vi "DriveGetModuleRef.vi"(11 "ModualNamePrefix":i32) -> (0 "SpinMot":T2, 1 "SpinStr":string, 2 "TravMot":T2, 3 "TravStr":string, 4 "EncStr":string, 5 "AbsEncoder":T1)   [LabVIEW 2025]
uses:
  <vilib>/Rock Robotics/SystemInterfaces/DIO/FPGA_DIOPWMChannel.ctl
  <vilib>/Rock Robotics/WPI/PWM/WPI_PWMDeadband.ctl
  <vilib>/Rock Robotics/WPI/MotorControl/WPI_MotorControlType.ctl
  <vilib>/Rock Robotics/SystemInterfaces/DIO/FPGA_DIOChannel.ctl
  <vilib>/Rock Robotics/WPI/MotorControl/WPI_MotorControlDeviceRef.ctl
  <vilib>/Rock Robotics/WPI/ThirdParty/Phoenix6/DeviceReference.ctl
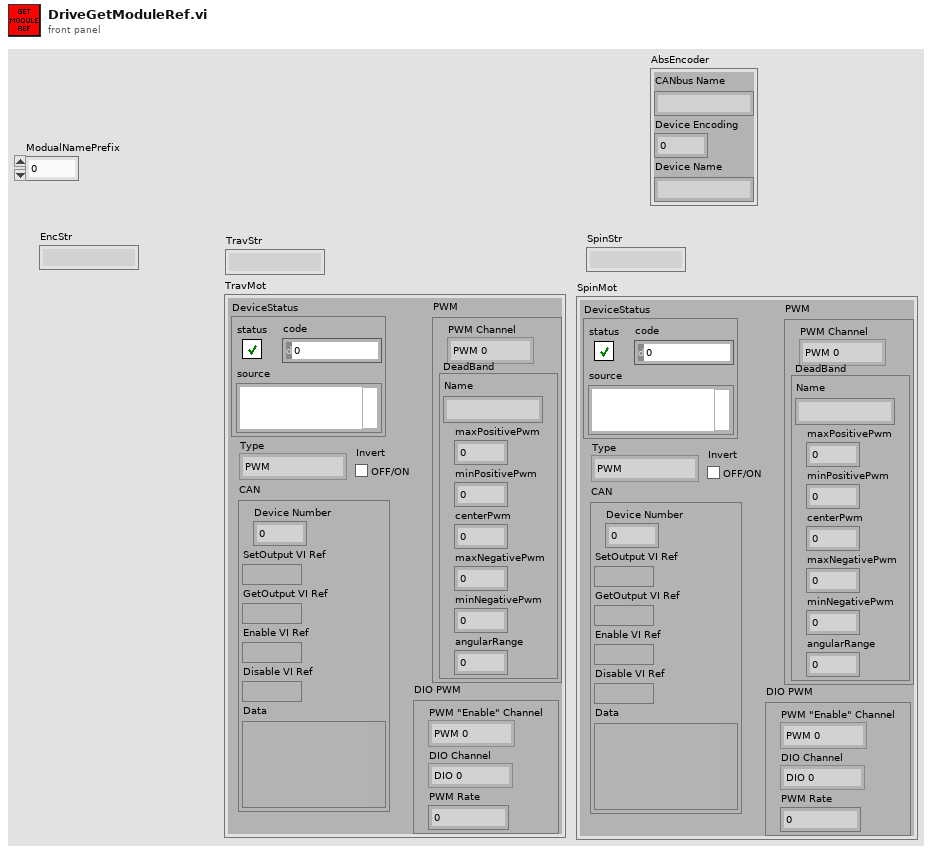
[diagram p1: front panel]
types:
  T1 = typedef "DeviceReference.ctl" = cluster{"CANbus Name":string, "Device Encoding":u32, "Device Name":string}
  T2 = typedef "WPI_MotorControlDeviceRef.ctl" = cluster{"DeviceStatus":errorcluster, "Type":T3, "PWM":cluster{"PWM Channel":T4, "DeadBand":T5}, "CAN":cluster{"Device Number":u8, "SetOutput VI Ref":variant, "GetOutput VI Ref":variant, "Enable VI Ref":variant, "Disable VI Ref":variant, "Data":variant}, "Invert":bool, "DIO PWM":cluster{"PWM \"Enable\" Channel":T4, "DIOChannel":T6, "PWM Rate":dbl}}
  T3 = typedef "WPI_MotorControlType.ctl" = enum16{"PWM", "CAN", "DIO PWM"}
  T4 = typedef "FPGA_DIOPWMChannel.ctl" = enum8{"PWM 0", "PWM 1", "PWM 2", "PWM 3", "PWM 4", "PWM 5", "PWM 6", "PWM 7", "PWM 8", "PWM 9", "PWM MXP 0", "PWM MXP 1", "PWM MXP 2", "PWM MXP 3", "PWM MXP 4", "PWM MXP 5", "PWM MXP 6", "PWM MXP 7", "PWM MXP 8", "PWM MXP 9", "Invalid"}
  T5 = typedef "WPI_PWMDeadband.ctl" = cluster{"Name":string, "maxPositivePwm":i32, "minPositivePwm":i32, "centerPwm":i32, "maxNegativePwm":i32, "minNegativePwm":i32, "angularRange":u16}
  T6 = typedef "FPGA_DIOChannel.ctl" = enum8{"DIO 0", "DIO 1", "DIO 2", "DIO 3", "DIO 4", "DIO 5", "DIO 6", "DIO 7", "DIO 8", "DIO 9", "DIO MXP 0", "DIO MXP 1", "DIO MXP 2", "DIO MXP 3", "DIO MXP 4", "DIO MXP 5", "DIO MXP 6", "DIO MXP 7", "DIO MXP 8", "DIO MXP 9", "DIO MXP 10", "DIO MXP 11", "DIO MXP 12", "DIO MXP 13", "DIO MXP 14", "DIO MXP 15", "SPI Port CS1", "SPI Port CS2", "SPI Port CS3", "SPI Port MISO", "SPI Port MOSI", "Invalid"}
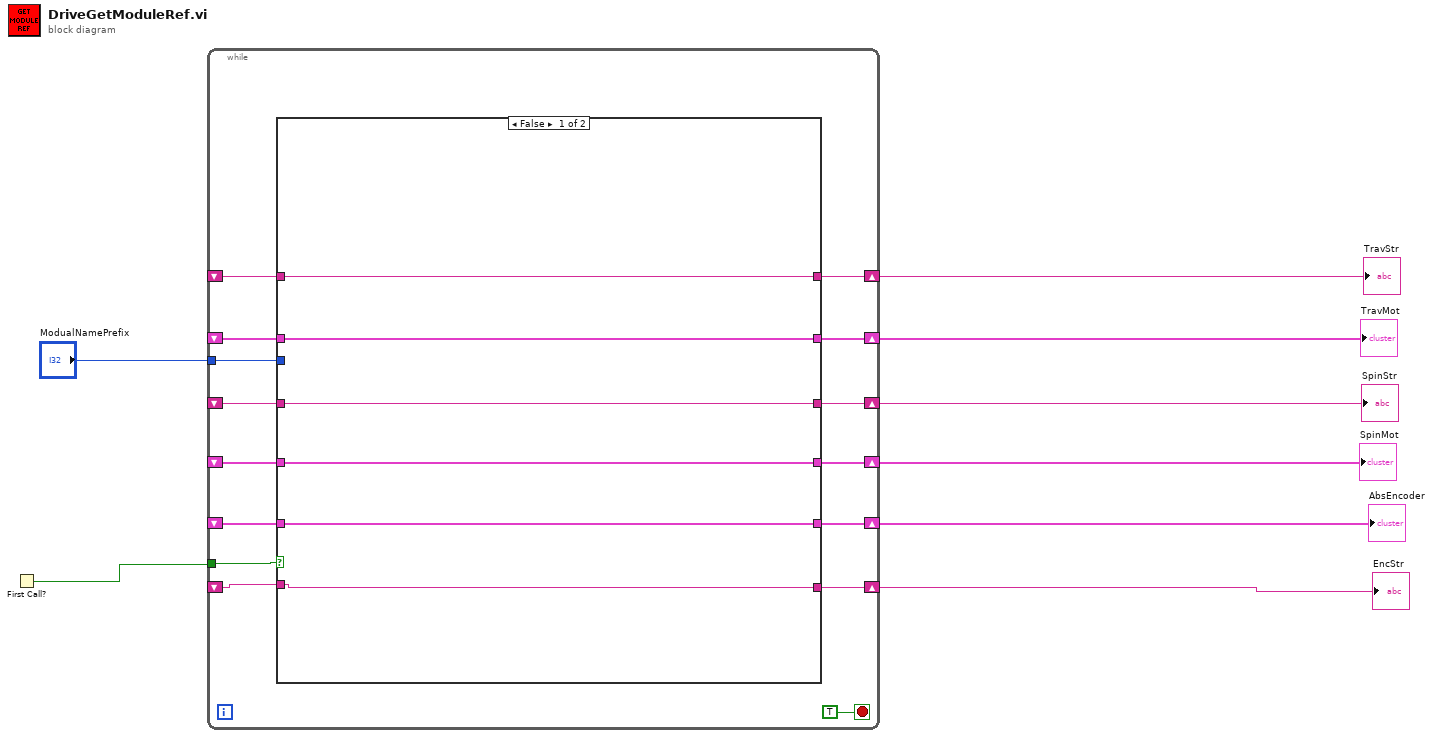
[diagram p0: block diagram]
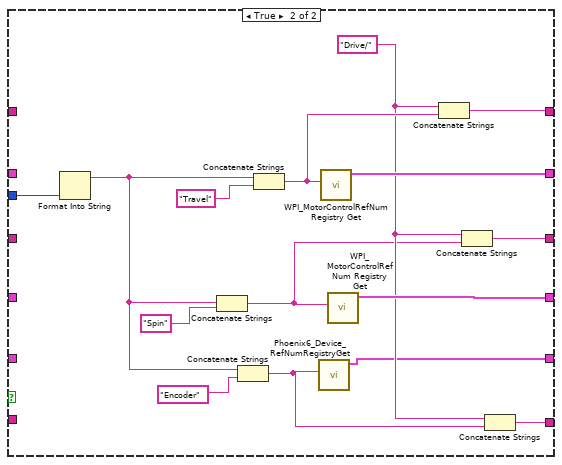
[diagram p2: hidden frame]
diagram:
  n1 = First Call?() -> (First Call?: T/F=w2:bool)
  n2 = while {
    tunnel: "ModualNamePrefix" -> [w23]
    tunnel: w2 -> [w17]
    shift-right: [w20] -> w5
    shift-left: _ -> [w15]
    shift-right: [w21] -> w6
    shift-left: _ -> [w14]
    shift-right: [w18] -> w3
    shift-left: _ -> [w13]
    shift-right: [w22] -> w7
    shift-left: _ -> [w12]
    shift-right: [w19] -> w4
    shift-left: _ -> [w11]
    shift-right: [w10] -> w1
    shift-left: _ -> [w9]
    stop <- TRUE stop-if-true
    n3 = case shown="False" w17 {
      tunnel: w23 -> [_ w44]
      tunnel: [w26 w42] -> w22
      tunnel: [w28 w41] -> w21
      tunnel: [w29 w36] -> w20
      tunnel: [w25 w35] -> w19
      tunnel: [w27 w33] -> w18
      tunnel: w15 -> [w29 _]
      tunnel: w14 -> [w28 _]
      tunnel: w13 -> [w27 _]
      tunnel: w12 -> [w26 _]
      tunnel: w11 -> [w25 _]
      tunnel: [w24 w30] -> w10
      tunnel: w9 -> [w24 _]
      frame False {
      }
      frame True {
        w34 = "Drive/" ("string")
        n4 = Format Into String(w44) -> (resulting string=w43:string)  [unwired: 3 in, 1 out]
        n5 = Concatenate Strings(w43, "Spin" ("refnum name")) -> (w32:string)
        n6 = Concatenate Strings(w43, "Encoder" ("refnum name")) -> (w31:string)
        n7 = Concatenate Strings(w43, "Travel" ("refnum name")) -> (w37:string)
        n8 = call <vilib>:"Phoenix6_Device_RefNumRegistryGet.vi"("refnum name"=w31) -> ("data"=w30:T1)  [unwired: 9 in, 1 out]
        n9 = call <vilib>:"WPI_MotorControlRefNum Registry Get.vi"("refnum name"=w37) -> ("MotorControlDevRef"=w41:T2)  [unwired: 9 in, 1 out]
        n10 = call <vilib>:"WPI_MotorControlRefNum Registry Get.vi"("refnum name"=w32) -> ("MotorControlDevRef"=w42:T2)  [unwired: 9 in, 1 out]
        n11 = Concatenate Strings(w34, w37) -> (w36:string)
        n12 = Concatenate Strings(w34, w32) -> (w33:string)
        n13 = Concatenate Strings(w34, w31) -> (w35:string)
      }
    }
  }
  "TravStr" <- w5
  "SpinStr" <- w3
  "SpinMot" <- w7
  "TravMot" <- w6
  "EncStr" <- w4
  "AbsEncoder" <- w1
